vi "Actor Core.vi"(8 "error in":errorcluster, 11 "HIJ File Viewer Demo App In":refnum<class "HIJ File Viewer Demo App.lvclass">) -> (0 "error out":errorcluster={"status"=FALSE, "code"=0, "source"="Actor Framework.lvlib:Actor.lvclass:Launch Nested Actor.vi<APPEND>\n\n<b>Complete call chain:</b>\r\n     Actor Framework.lvlib:Actor.lvclass:Launch Nested Actor.vi\r\n     Launch HIJ FileViewer.lvlib:Launch File Viewer.lvclass:Actor Core.vi"}, 3 "Actor out":refnum<class "Actor.lvclass">)   [LabVIEW 2014, in "HIJ File Viewer Demo App.lvlib" / "HIJ File Viewer Demo App.lvclass"]
doc: "(<B>Filename</B>: Actor Framework.lvlib:Actor.lvclass:Actor Core.vi)\n\nReceives messages to the actor, reacts to them, and initiates any error handling that may shut the actor down.\n\nDescendant classes may override this VI to append parallel tasks for the actor to complete while it handles messages. Overrides use the Call Parent Method node."
uses:
  HIJ File Viewer Demo App.lvclass
  <vilib>/ActorFramework/Actor/Actor.lvclass
  Applications/Launch HIJ FileViewer/HIJ Vision File Viewer App/HIJ Vision File Viewer App.lvclass
  Analyze/Analyze Classes/Analyze Diviation/Analyze BeamDeviation.lvclass
  Analyze/Results and Overlays/Results Beam Deviation/Analyze Results Beam Deviation.lvclass
  Analyze/Analyze Classes/Analyze Distanz/Analyze Distanz.lvclass
  Analyze/Results and Overlays/Results Distance/Analyze Results Distanz.lvclass
  Analyze/Analyze Classes/Analyze Fluence/Analyze Fluence.lvclass
  Analyze/Results and Overlays/Results Fluence/Analyze Results Fluence.lvclass
  Analyze/Analyze Parameter/Analyze Parameter Energy/Analyze Parameter Energy.lvclass
  Analyze/Analyze Parameter/Analyze Parameter Fluence/Analyze Parameter Fluence.lvclass
  Analyze/Analyze Classes/Analyze Total Counts/Analyze Total Counts.lvclass
  Analyze/Results and Overlays/Results Total Counts/Analyze Results Total Counts.lvclass
  Analyze/Analyze Parameter/Analyze Parameter Energy/Analyze Parameter Energy.lvclass/Analyze Parameter Energy.ctl
  Analyze/Results and Overlays/Results Fluence/Analyze Results Fluence.lvclass/Analyze Results Fluence.ctl
  Analyze/Results and Overlays/Results Total Counts/Analyze Results Total Counts.lvclass/Analyze Results Total Counts.ctl
  Applications/HIJ Vision Application/HIJ Vision Application/HIJ Vision Application.lvclass/HIJ Vision Application.ctl
  <vilib>/ActorFramework/Actor/Actor.lvclass/Actor.ctl
  <vilib>/ActorFramework/Message Enqueuer/Message Enqueuer.lvclass/Message Enqueuer.ctl
  Shared Code/Viewable Actor/ViewableActor Messages/Insert Into SubPanel Msg/Insert Into SubPanel Msg.lvclass/Insert Into SubPanel Msg.ctl
  Applications/HIJ Vision Application/HIJ Vision Application Messages/Set Parameter Msg/Set Parameter Msg.lvclass/Set Parameter Msg.ctl
  Analyze/Analyze Parameter/Analyze Parameter Energy/Write Energy.vi
  Analyze/Results and Overlays/Results Total Counts/Write UI Ref Total Counts.vi
  Analyze/Results and Overlays/Results Fluence/Write UI Ref Max F.vi
  Applications/HIJ Vision Application/HIJ Vision Application/Write Analyze Objs.vi
  <vilib>/ActorFramework/Message Enqueuer/Init from Existing Queue.vi
  <vilib>/ActorFramework/Message Enqueuer/Enqueue.vi
  <vilib>/ActorFramework/Message Priority Queue/Priority Enqueue.vi
  <vilib>/ActorFramework/Message Enqueuer/Message Enqueuer.lvclass
  Shared Code/Viewable Actor/ViewableActor Messages/Insert Into SubPanel Msg/Insert Into SubPanel Msg.lvclass
  Applications/HIJ Vision Application/HIJ Vision Application Messages/Set Parameter Msg/Set Parameter Msg.lvclass
  <vilib>/ActorFramework/Stop Msg/Stop Msg.lvclass
panel:
  in  "Stop Button":bool=TRUE
  out "Total Counts":dbl=20.0 format="%#.2g"
  out "Max F":dbl[unit]=200000.0 format="%#.2g"
  in  "Energy":dbl[unit]=20.0 format="%#_13g"
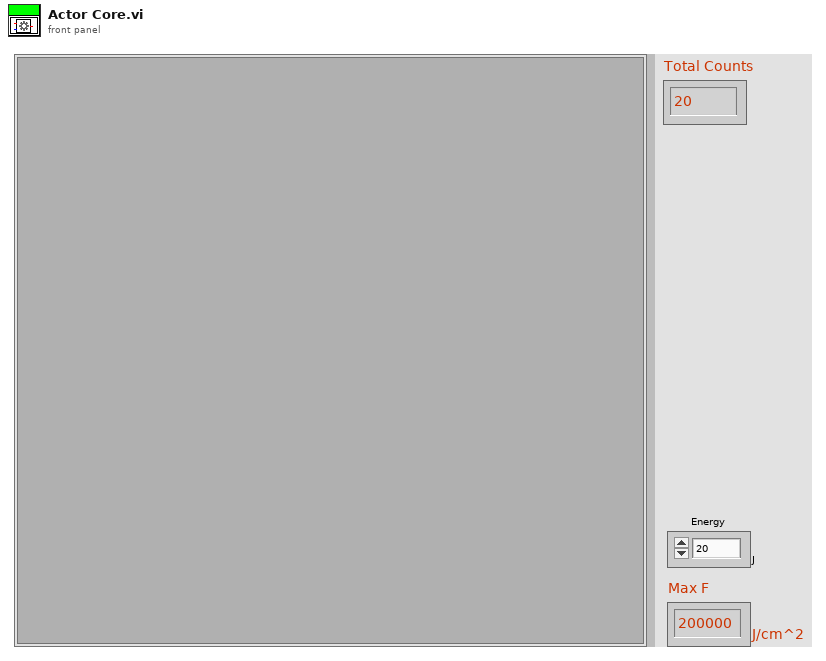
[diagram p1: front panel]
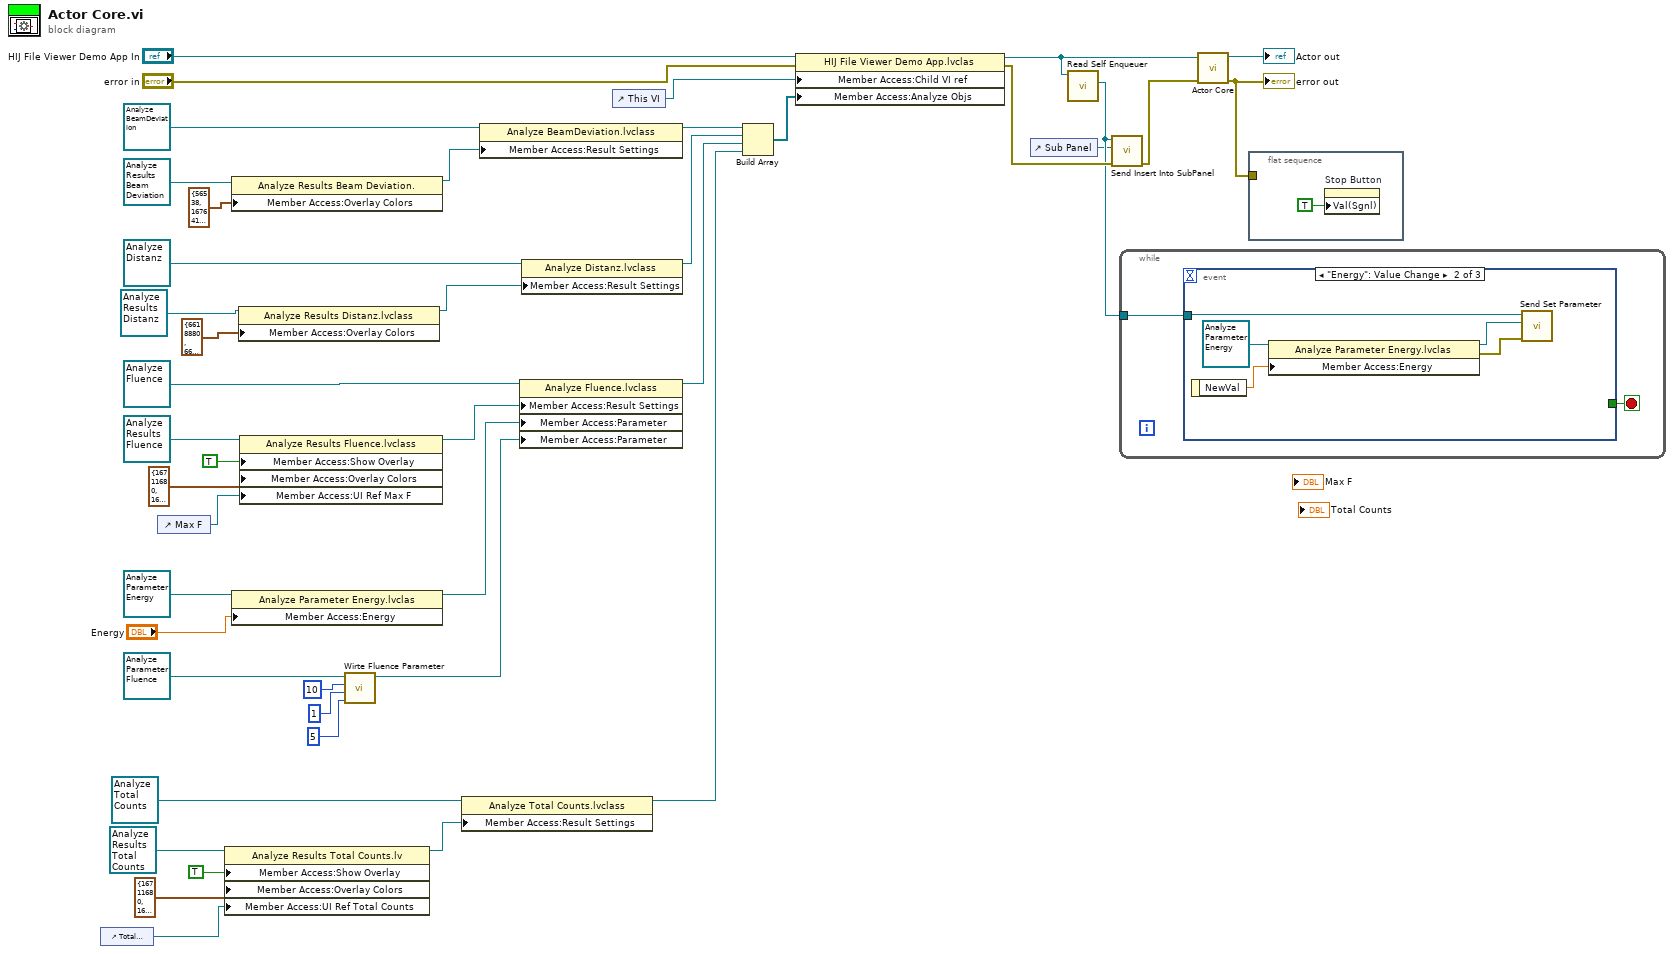
[diagram p0: block diagram]
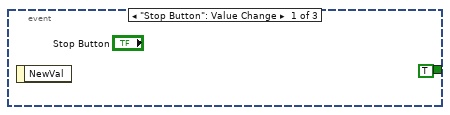
[diagram p2: hidden frame]
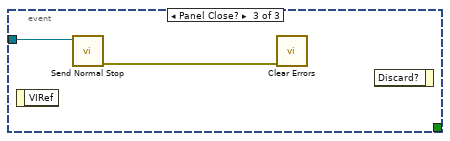
[diagram p3: hidden frame]
diagram:
  n1 = control-ref of="Total Counts"() -> (w2:refnum<vi>)
  n2 = control-ref of="Max F"() -> (w15:refnum<vi>)
  n3 = property class="Analyze Results Total Counts.lv"(reference=refnum<class "Analyze Results Total Counts.lvclass"> refnum ("Analyze Results Total Counts.lvclass"), "Member Access:Show Overlay"=TRUE ("bOverlay"), "Member Access:Overlay Colors"=cluster{"Border":u32, "Text":u32} {"Border"=16711680, "Text"=16448250} ("Colors"), "Member Access:UI Ref Total Counts"=w2) -> (reference out=w3:refnum<class "Analyze Results Total Counts.lvclass">)  [unwired: 1 in, 1 out]
  n4 = property class="Analyze Results Beam Deviation."(reference=refnum<class "Analyze Results Beam Deviation.lvclass"> refnum ("Analyze Results Beam Deviation.lvclass"), "Member Access:Overlay Colors"=cluster{"Border":u32, "Text":u32} {"Border"=56538, "Text"=16764160} ("Colors")) -> (reference out=w28:refnum<class "Analyze Results Beam Deviation.lvclass">)  [unwired: 1 in, 1 out]
  n5 = property class="Analyze Parameter Energy.lvclas"(reference=refnum<class "Analyze Parameter Energy.lvclass"> refnum ("Analyze Parameter Energy.lvclass"), "Member Access:Energy"="Energy") -> (reference out=w25:refnum<class "Analyze Parameter Energy.lvclass">)  [unwired: 1 in, 1 out]
  n6 = property class="Analyze Results Distanz.lvclass"(reference=refnum<class "Analyze Results Distanz.lvclass"> refnum ("Analyze Results Distanz.lvclass"), "Member Access:Overlay Colors"=cluster{"Border":u32, "Text":u32} {"Border"=6618880, "Text"=6618880} ("Colors")) -> (reference out=w27:refnum<class "Analyze Results Distanz.lvclass">)  [unwired: 1 in, 1 out]
  n7 = property class="Analyze Results Fluence.lvclass"(reference=refnum<class "Analyze Results Fluence.lvclass"> refnum ("Analyze Results Fluence.lvclass"), "Member Access:Show Overlay"=TRUE ("bOverlay"), "Member Access:Overlay Colors"=cluster{"Border":u32, "Text":u32} {"Border"=16711680, "Text"=16448250} ("Colors"), "Member Access:UI Ref Max F"=w15) -> (reference out=w30:refnum<class "Analyze Results Fluence.lvclass">)  [unwired: 1 in, 1 out]
  n8 = call "Wirte Fluence Parameter.vi"("#of Areas"=5, "#Overlays"=1, "Size of region (px)"=10, "Analyze Parameter Fluence in"=refnum<class "Analyze Parameter Fluence.lvclass"> refnum ("Analyze Parameter Fluence.lvclass")) -> ("Analyze Parameter Fluence out"=w23:refnum<class "Analyze Parameter Fluence.lvclass">)  [unwired: 7 in]
  n9 = property class="Analyze Total Counts.lvclass"(reference=refnum<class "Analyze Total Counts.lvclass"> refnum ("Analyze.lvlib:Analyze Total Counts.lvclass"), "Member Access:Result Settings"=w3) -> (reference out=w1:refnum<class "Analyze Total Counts.lvclass">)  [unwired: 1 in, 1 out]
  n10 = property class="Analyze BeamDeviation.lvclass"(reference=refnum<class "Analyze BeamDeviation.lvclass"> refnum ("Analyze.lvlib:Analyze BeamDeviation.lvclass"), "Member Access:Result Settings"=w28) -> (reference out=w29:refnum<class "Analyze BeamDeviation.lvclass">)  [unwired: 1 in, 1 out]
  n11 = property class="Analyze Fluence.lvclass"(reference=refnum<class "Analyze Fluence.lvclass"> refnum ("Analyze.lvlib:Analyze Fluence.lvclass"), "Member Access:Result Settings"=w30, "Member Access:Parameter"=w25, "Member Access:Parameter"=w23) -> (reference out=w18:refnum<class "Analyze Fluence.lvclass">)  [unwired: 1 in, 1 out]
  n12 = property class="Analyze Distanz.lvclass"(reference=refnum<class "Analyze Distanz.lvclass"> refnum ("Analyze.lvlib:Analyze Distanz.lvclass"), "Member Access:Result Settings"=w27) -> (reference out=w19:refnum<class "Analyze Distanz.lvclass">)  [unwired: 1 in, 1 out]
  n13 = control-ref of="This VI"() -> (w8:refnum<vi>)
  n14 = Build Array(w29, w19, w18, w1) -> (w9:refnum<class "Analyze BaseClass.lvclass">[])
  n15 = property class="HIJ File Viewer Demo App.lvclas"(reference="HIJ File Viewer Demo App In", error in="error in", "Member Access:Child VI ref"=w8, "Member Access:Analyze Objs"=w9) -> (reference out=w10:refnum<class "HIJ File Viewer Demo App.lvclass">, error out=w14:errorcluster)
  n16 = control-ref of="Sub Panel"() -> (w11:refnum<vi>)
  n17 = call <vilib>:"Read Self Enqueuer.vi"("Actor"=w10) -> ("Self Enqueuer"=w12:refnum<class "Message Enqueuer.lvclass">)  [unwired: 10 in]
  n18 = call "Send Insert Into SubPanel.vi"("error in (no error)"=w14, "SubPanel Ref"=w11, "Message Enqueuer"=w12) -> ("error out"=w13:errorcluster)  [unwired: 7 in, 1 out]
  n19 = while {
    tunnel: w12 -> [w44]
    stop <- w45 stop-if-true
    n20 = event shown="[1] \"Energy\": Value Change" {
      selector: _ -> [_ _ _]
      dyn-events: _ -> [_ _ _]
      timeout: _ -> [_ _ _]
      tunnel: [TRUE _ _] -> w45
      tunnel: w44 -> [_ w51 w53]
      event "Stop Button": Value Change {
        n21 = event-data() -> ()  [unwired: 1 in, 1 out]
      }
      event "Energy": Value Change {
        n22 = event-data() -> ("NewVal"=w48:dbl[unit])  [unwired: 1 in]
        n23 = property class="Analyze Parameter Energy.lvclas"(reference=refnum<class "Analyze Parameter Energy.lvclass"> refnum ("Analyze Parameter Energy.lvclass"), "Member Access:Energy"=w48) -> (reference out=w47:refnum<class "Analyze Parameter Energy.lvclass">, error out=w49:errorcluster)  [unwired: 1 in]
        n24 = call "Send Set Parameter.vi"("error in (no error)"=w49, "Parameter"=w47, "Message Enqueuer"=w51) -> ()  [unwired: 7 in, 2 out]
      }
      event Panel Close? {
        n25 = event-data() -> ()  [unwired: 1 in, 1 out]
        n26 = call <vilib>:"Send Normal Stop.vi"("Message Enqueuer"=w53) -> ("error out"=w52:errorcluster)  [unwired: 10 in]
        n27 = call <vilib>:"Clear Errors.vi"("error in (no error)"=w52) -> ()  [unwired: 5 in, 2 out]
        n28 = event-data() -> ()  [unwired: 2 in, 1 out]
      }
    }
  }
  n29 = call-parent "Actor Core.vi"("error in"=w13, "Launch IMAQ Display in"=w10) -> ("error out"=w16:errorcluster, "Actor out"=→"Actor out":refnum<class "Actor.lvclass">)  [unwired: 8 in]
  "error out" <- w16
  n30 = flat-sequence {
    tunnel: w16 -> [_]
    frame #0 {
      n31 = property on="Stop Button" class="Bool (strict)"("Val(Sgnl)"=TRUE) -> ()  [unwired: 2 in, 2 out]
    }
  }
